vi "Open_File_for_Read.vi"(11 "file path":path) -> (0 "error out":errorcluster, 1 "exists?":bool, 2 "Permission error?":bool, 3 "refnum":refnum<file>)   [LabVIEW 2020]
doc: "Opens an existing file, creates a new file, or replaces an existing file, programmatically or interactively using dialog. You can optionally specify a dialog prompt, default file name, start path, or filter pattern, and you can specify open and deny modes when opening a file, plus group and permission when creating a new file. Use this VI with the intermediate Write File+ or Read File+ VIs described below.\n\nfile path is the path name of the file. If file path is empty (default value) or is Not A Path, the VI displays a File dialog box from which you can select a file. Error 43 occurs if the user cancels the dialog. \n\nfunction is the operation to perform:\n\n 0 (open) opens an existing file. Error 7 occurs if the file cannot be found.\n \n 1 (open or create) opens an existing file or creates a new file if one does not exist.\n\n 2 (create or replace) creates a new file or replaces a file if it exists and you give permission. Replacement is done by opening the file and setting EOF to 0. Error 43 occurs if the user elects to disallow the replacement using dialog. \n\n 3 (create) creates a new file. Error 8 occurs if the file already exists.\n\nadvisory dialog? Set TRUE (default) if you want a dialog if function=0 and the file does not exist, or if function=2 or 3 and the file exists.\n\nprompt is the message that appears below the list of files and directories in the file dialog.\n\ndefault name is the initial file name that appears in the selection box of the file dialog.\n\nstart path is the path name to the initially displayed directory in a file dialog. The default value is Not A Path, which is the path to the last directory shown in a file dialog.\n\npattern is the match pattern specification to display only certain types of files or directories. See the description of the File Dialog function for more information.\n\nerror in is a cluster of three elements (error?, code, and source) that describe the upstream error state, that is, the existance of any error preceeding the execution of the VI. The VI executes normally only if no incoming error exists; otherwise it merely passes the error in value to error out. error? is TRUE if an error occurred; the default value is FALSE. code is the error code; the default value is 0. source is in most cases the name of the VI or function that produced the error; the default value is an empty string.\n\nnew file path is the path of the file opened or created. You can use this output to determine the path of a file that you open or create using dialog. new file path returns Not A Path if the user selects Cancel from the dialog box.\n\nrefnum is the reference number of the open file. The value is Not A Refnum if the file cannot be opened.\n\nfile size is the size of the file in bytes; it is also the location of the end of file.\n\nerror out is a cluster of three elements (error?, code, and source) that describe the error state following the execution of the VI. If an incoming error does not exist, the VI executes normally and error out describes the VI's error state; if an incoming error exists, error out equals error in."
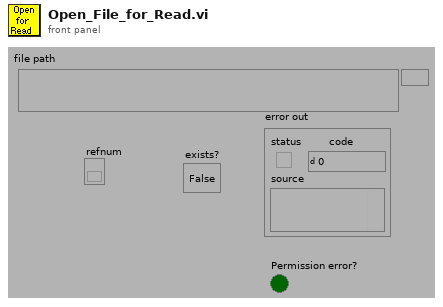
[diagram p1: front panel]
types:
  T1 = enum16{"open", "replace", "create", "open or create", "replace or create", "replace or create with confirmation"}
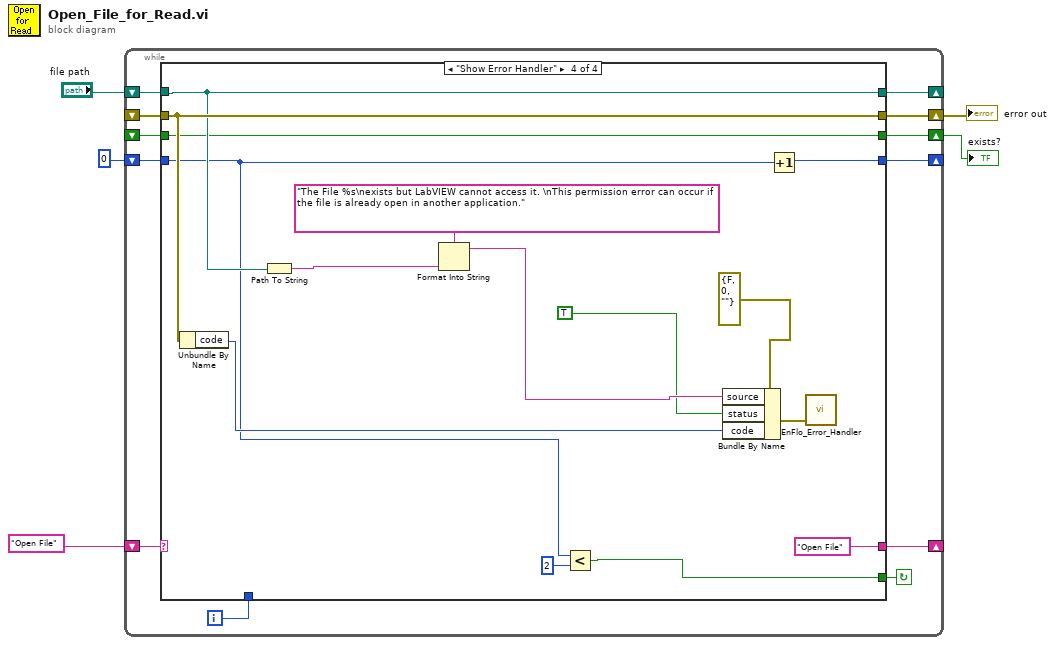
[diagram p0: block diagram]
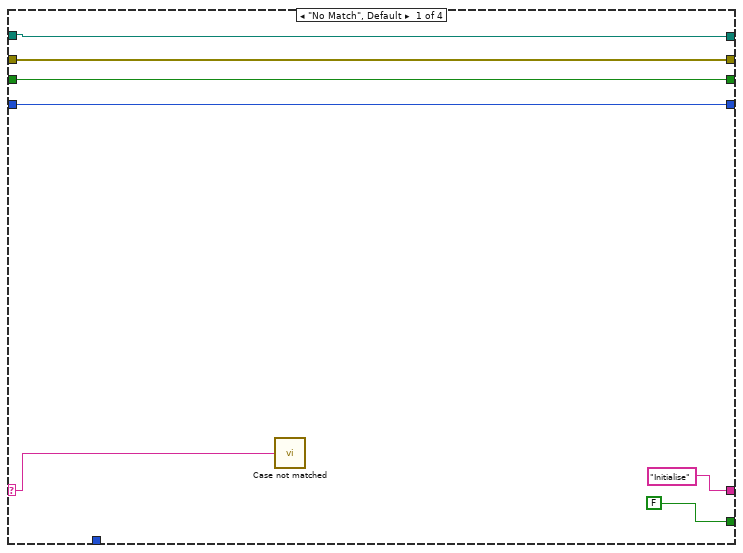
[diagram p2: hidden frame]
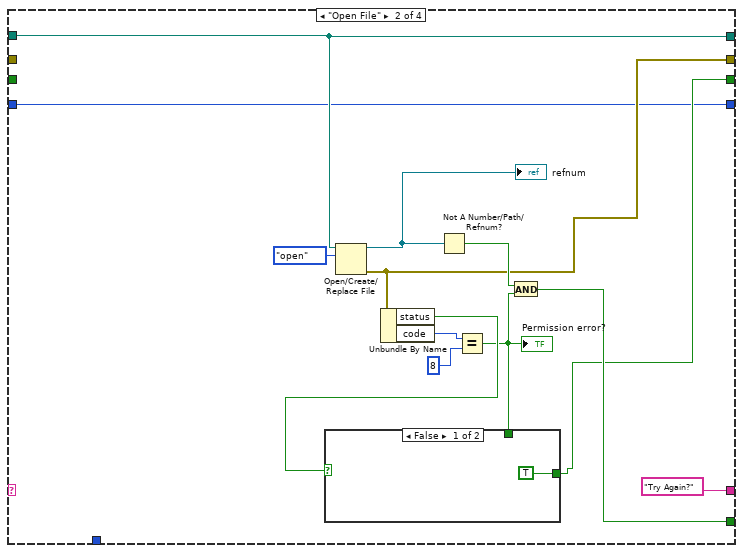
[diagram p3: hidden frame]
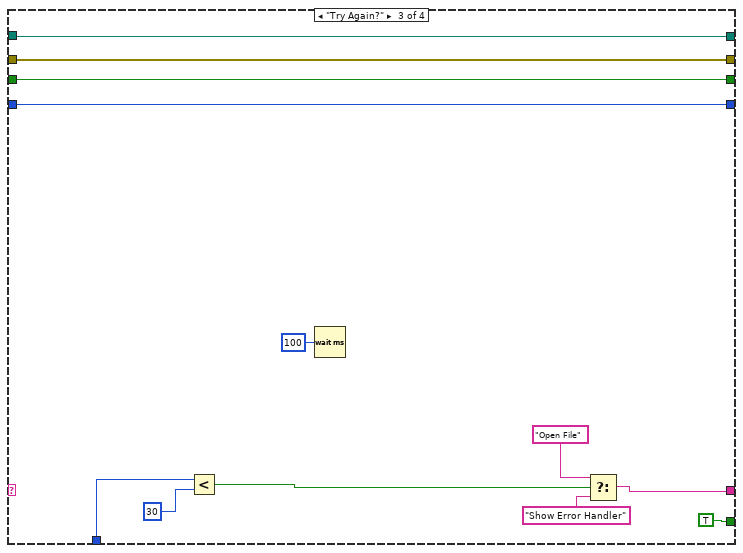
[diagram p5: hidden frame]
diagram:
  n1 = while {
    shift-left: "Open File" -> [w15]
    shift-right: [w16] -> _
    shift-right: [w13] -> w4
    shift-left: _ -> [w10]
    shift-right: [w11] -> _
    shift-left: "file path" -> [w12]
    shift-right: [w8] -> w2
    shift-left: _ -> [w9]
    shift-right: [w6] -> _
    shift-left: 0 -> [w7]
    i -> [w14]
    stop <- w17 continue-if-true
    n2 = case shown="\"Show Error Handler\"" w15 {
      selector: w15 -> [w18 _ _ _]
      tunnel: [FALSE w31 TRUE w54] -> w17
      tunnel: ["Initialise" "Try Again?" w46 "Open File"] -> w16
      tunnel: w12 -> [w22 w36 w42 w65]
      tunnel: w14 -> [_ _ w49 _]
      tunnel: [w21 w30 w43 w66] -> w13
      tunnel: [w22 w36 w42 w65] -> w11
      tunnel: w10 -> [w21 _ w43 w66]
      tunnel: w9 -> [w20 _ w41 w57]
      tunnel: [w20 w27 w41 w57] -> w8
      tunnel: w7 -> [w19 w26 w40 w53]
      tunnel: [w19 w26 w40 w52] -> w6
      frame "No Match", Default {
        n3 = call "Case not matched.vi"("Case Name not Matched"=w18) -> ()
      }
      frame "Open File" {
        n4 = Open/Create/Replace File(file path (use dialog)=w36, operation (0:open)=T1."open") -> (refnum out=w35:refnum<file>, error out=w30:errorcluster)  [unwired: 2 in, 3 out]
        "refnum" <- w35
        n5 = Unbundle By Name(w30) -> ("status"=w29:bool, "code"=w34:i32)
        n6 = Not A Number/Path/Refnum?(number/path/refnum=w35) -> (NaN/Path/Refnum?=w32:bool)
        n7 = Equal?(x=w34, y=8) -> (x = y?=w28:bool)
        "Permission error?" <- w28
        n8 = case shown="False" w29 {
          tunnel: [TRUE w39] -> w27
          tunnel: w28 -> [_ w39]
          frame False {
          }
          frame True {
          }
        }
        n9 = And(x=w32, y=w28) -> (x .and. y?=w31:bool)
      }
      frame "Try Again?" {
        n10 = Less?(x=w49, y=30) -> (x < y?=w47:bool)
        n11 = Wait (ms)(milliseconds to wait=u32 100) -> ()  [unwired: 1 out]
        n12 = Select(t="Open File", s=w47, f="Show Error Handler") -> (s? t:f=w46:string)
      }
      frame "Show Error Handler" {
        n13 = Unbundle By Name(w66) -> ("code"=w61:i32)
        n14 = Path To String(path=w65) -> (string=w58:string)
        n15 = Format Into String(format string="The File %s\nexists but LabVIEW cannot access it. \nThis permission error can occur if the file is already open in another application." ("Format String"), w58) -> (resulting string=w62:string)  [unwired: 2 in, 1 out]
        n16 = Less?(x=w53, y=2) -> (x < y?=w54:bool)
        n17 = Bundle By Name(cluster=errorcluster {"status"=FALSE, "code"=0, "source"=""} ("error in (no error)"), "source"=w62, "status"=TRUE, "code"=w61) -> (w64:errorcluster)
        n18 = Increment(x=w53) -> (x+1=w52:i32)
        n19 = call "EnFlo_Error_Handler.vi"("error in (no error)"=w64) -> ()  [unwired: 2 in, 3 out]
      }
    }
  }
  "error out" <- w4
  "exists?" <- w2
